vi "Forensic_Snapshot.vi"(9 "Declencher":bool, 10 "Dossier Forensics":path, 11 "Fichier log":path) -> (2 "Chemin snapshot":path, 3 "Snapshot cree":bool)   [LabVIEW 2022 SP3]
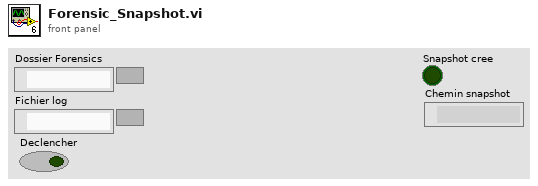
[diagram p1: front panel]
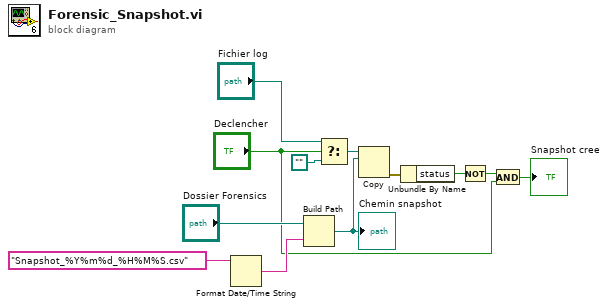
[diagram p0: block diagram]
diagram:
  n1 = Format Date/Time String(time format string (%c)="Snapshot_%Y%m%d_%H%M%S.csv") -> (date/time string=w12:string)  [unwired: 2 in]
  n2 = Build Path(base path="Dossier Forensics", name or relative path=w12) -> (appended path=w11:path)
  "Chemin snapshot" <- w11
  n3 = Select(t="Fichier log", s="Declencher", f=path "") -> (s? t:f=w10:path)
  n4 = Copy(10:w11, 11:w10) -> (0:w9:errorcluster)  [unwired: 3 in, 2 out]
  n5 = Unbundle By Name(w9) -> ("status"=w6:bool)
  n6 = Not(x=w6) -> (.not. x?=w8:bool)
  n7 = And(x=w8, y="Declencher") -> (x .and. y?=→"Snapshot cree":bool)
